vi "Add Initialization Block Diagram Content.vi"(8 "error in (no error)":errorcluster, 10 "Init":T1, 11 "Module in":refnum<class "Module.lvclass">) -> (0 "error out":errorcluster, 3 "Module out":refnum<class "Module.lvclass">)   [LabVIEW 2015, in "Module.lvclass"]
uses:
  Module.lvclass
  Loop/Block Diagram/Init.Refs.ctl
  <vilib>/Utility/miscctls.llb/LVPointTypeDef.ctl
  Module.lvclass/Module.ctl
  IO/IO Class/Signal.lvclass
  Loop/Block Diagram/Block Diagram.lvclass
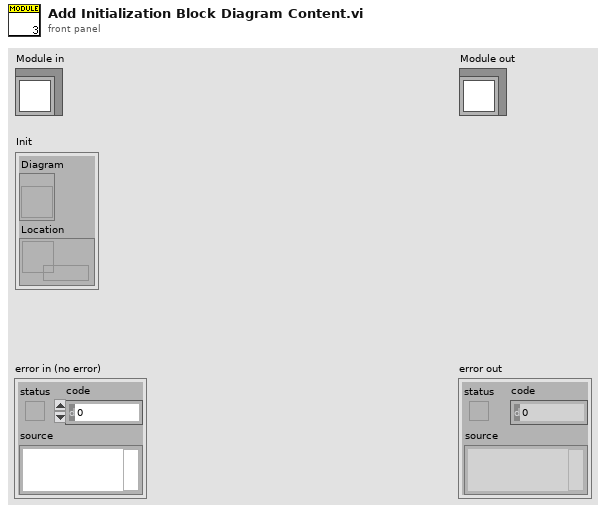
[diagram p1: front panel]
types:
  T1 = typedef "Block Diagram.lvclass/Init.Refs.ctl" = cluster{"Diagram":refnum<vi>, "Location":refnum<data-value>}
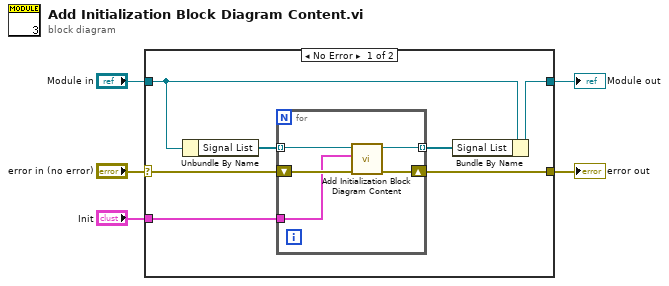
[diagram p0: block diagram]
diagram:
  n1 = case shown="No Error" "error in (no error)" {
    selector: "error in (no error)" -> [w8 w19]
    tunnel: [w11 w19] -> w4
    tunnel: [w9 w18] -> w2
    tunnel: "Module in" -> [w7 w18]
    tunnel: "Init" -> [w12 _]
    frame No Error {
      n2 = Unbundle By Name(w7) -> ("Signal List"=w6:refnum<class "Signal.lvclass">[])
      n3 = for {
        shift-right: [w16] -> w11
        shift-left: w8 -> [w17]
        tunnel: w12 -> [w15]
        tunnel: [w14] -> w10 mode=indexing
        tunnel: w6 -> [w13] mode=indexing
        n4 = call-dynamic "Add Initialization Block Diagram Content.vi"("error in (no error)"=w17, "Init"=w15, "IO Class in"=w13) -> ("error out"=w16:errorcluster, "IO Class out"=w14:refnum<class "Signal.lvclass">)  [unwired: 7 in]
      }
      n5 = Bundle By Name(cluster=w7, "Signal List"=w10) -> (w9:refnum<class "Module.lvclass">)
    }
    frame Error {
    }
  }
  "error out" <- w4
  "Module out" <- w2
